vi "UpdateConfig.vi"(8 "Error In":errorcluster, 10 "TestSettings":T1, 11 "AutoData":T2) -> (0 "Error Out":errorcluster, 3 "AutoData out":T2)   [LabVIEW 2019, in "AutoMode.lvlib"]
uses:
  AutoMode.lvlib
  Cluster - AutoModeData.ctl
  MainController/Cluster - TestSettings.ctl
  MainController/Cluster - HardwareConfiguration.ctl
  MainController/Cluster - TestResults.ctl
  Cluster - AutoModeMessage.ctl
  Enum - AutoModeState.ctl
  MainController/Cluster - MainControllerMessage.ctl
  MainController/Enum - MainState.ctl
  MainController/MainController.lvlib
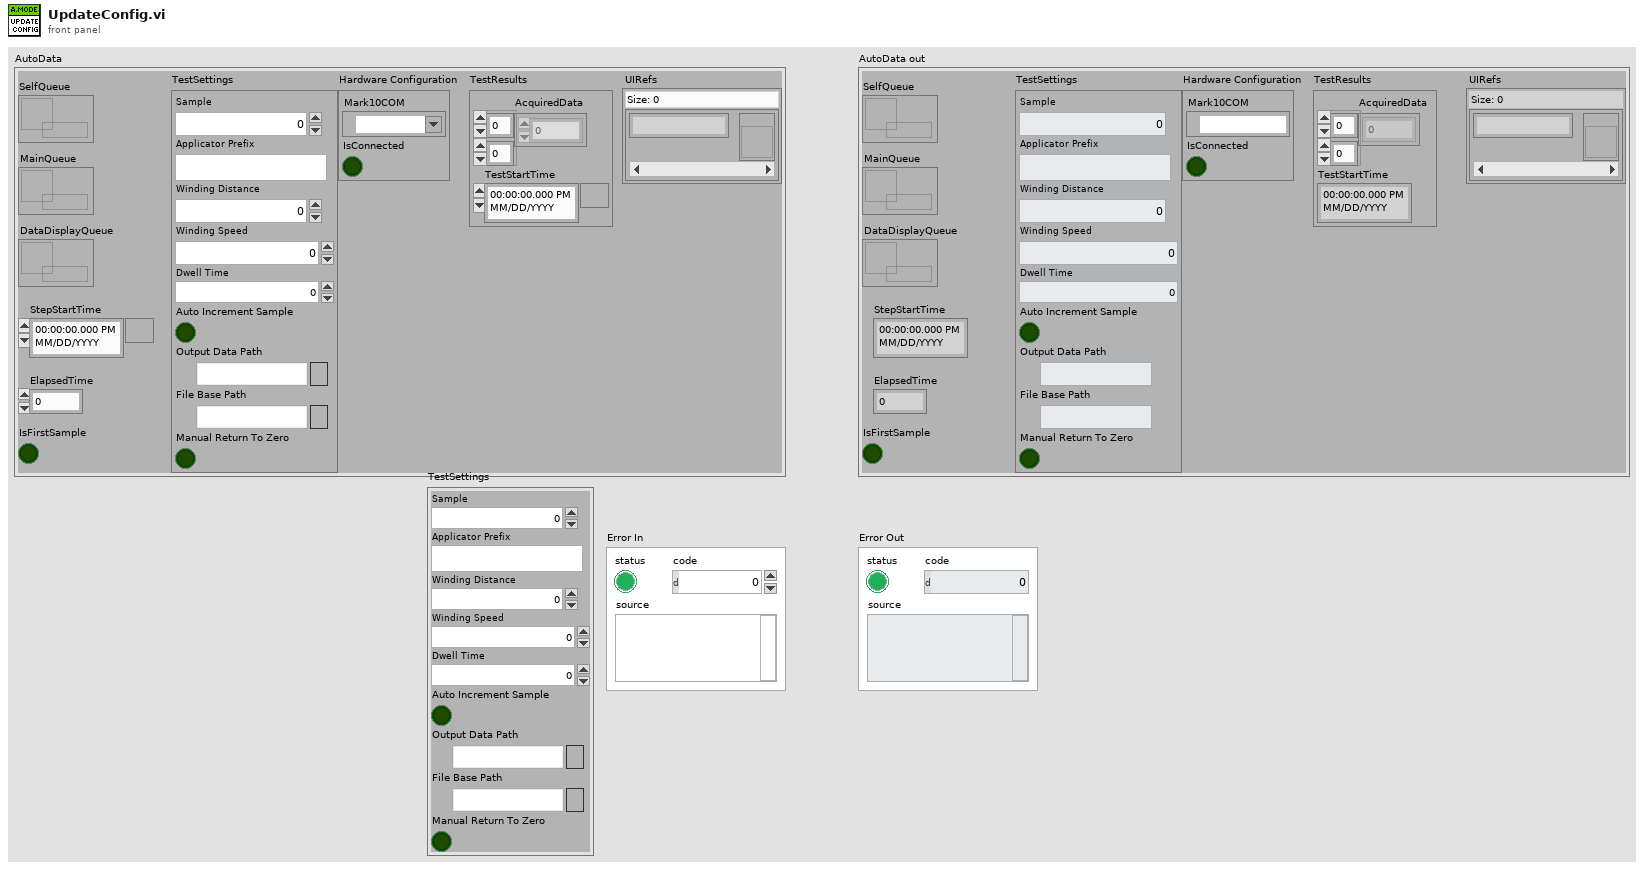
[diagram p1: front panel]
types:
  T1 = typedef "MainController.lvlib/Cluster - TestSettings.ctl" = cluster{"Sample":u32, "Applicator Prefix":string, "Winding Distance":dbl, "Winding Speed":dbl, "Dwell Time":dbl, "Auto Increment Sample":bool, "Output Data Path":path, "File Base Path":path, "Manual Return To Zero":bool}
  T2 = typedef "AutoMode.lvlib/Cluster - AutoModeData.ctl" = cluster{"DataDisplayQueue":refnum<queue>, "StepStartTime":timestamp, "TestSettings":T1, "Hardware Configuration":T3, "TestResults":T4, "ElapsedTime":dbl, "IsFirstSample":bool, "SelfQueue":refnum<queue>, "MainQueue":refnum<queue>, "UIRefs":map{string, refnum<vi>}}
  T3 = typedef "MainController.lvlib/Cluster - HardwareConfiguration.ctl" = cluster{"Mark10COM":refnum<visa-resource-name>, "IsConnected":bool}
  T4 = typedef "MainController.lvlib/Cluster - TestResults.ctl" = cluster{"AcquiredData":dbl[][], "TestStartTime":timestamp}
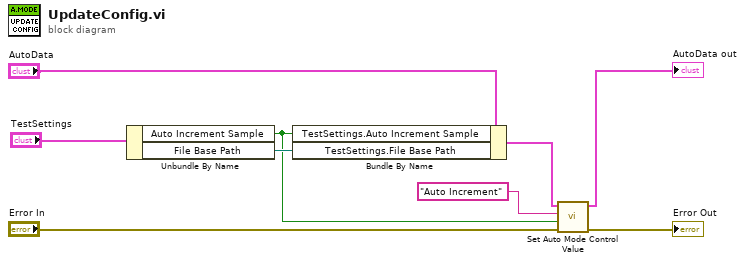
[diagram p0: block diagram]
diagram:
  n1 = Unbundle By Name("TestSettings") -> ("Auto Increment Sample"=w1:bool, "File Base Path"=w7:path)
  n2 = Bundle By Name(cluster="AutoData", "TestSettings.Auto Increment Sample"=w1, "TestSettings.File Base Path"=w7) -> (w4:T2)
  n3 = call "Set Auto Mode Control Value.vi"("Error In"="Error In", "Value"=w1, "key"="Auto Increment", "AutoData"=w4) -> ("Error Out"=→"Error Out":errorcluster, "AutoData out"=→"AutoData out":T2)  [unwired: 6 in]
